vi "Fault States to Word.vi"(11 "Fault States":T1[](array[typedef])) -> (3 "Fault Word":u16 format="%016b")   [LabVIEW 2014, in "SLSC configuration Shared.lvlib"]
doc: "Converts four faults to a fault word."
uses:
  SLSC configuration Shared.lvlib
  Fault State.ctl
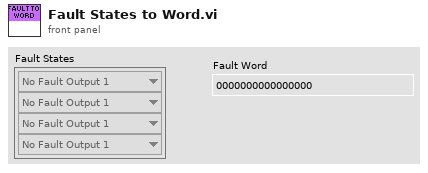
[diagram p1: front panel]
types:
  T1 = typedef "SLSC configuration Shared.lvlib/Fault State.ctl" = enum8{"No Fault Output 1", "Open Circuit 100 Hz", "Ground 100 Hz", "Open Circuit", "Ground", "Fail Rail 1", "Fail Rail 2", "No Fault Output 2"}
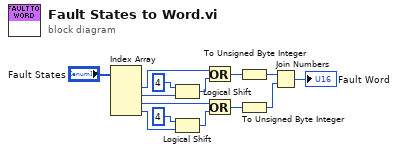
[diagram p0: block diagram]
diagram:
  n1 = Index Array(array="Fault States") -> (element #1=w9:T1, element #2=w11:T1, element #3=w6:T1, element #4=w12:T1)  [unwired: 4 in]
  n2 = Logical Shift(y=u16 4, x=w11) -> (x << y=w8:u32)
  n3 = Logical Shift(y=u16 4, x=w12) -> (x << y=w7:u32)
  n4 = Or(x=w9, y=w8) -> (x .or. y?=w5:u32)
  n5 = Or(x=w6, y=w7) -> (x .or. y?=w4:u32)
  n6 = To Unsigned Byte Integer(number=w5) -> (unsigned 8bit integer=w3:u8)
  n7 = To Unsigned Byte Integer(number=w4) -> (unsigned 8bit integer=w2:u8)
  n8 = Join Numbers(hi=w3, lo=w2) -> ((hi.lo)=→"Fault Word":u16)
